vi "Get Standard VI Data.vi"(8 "error in (no error)":errorcluster, 11 "VI Ref":refnum<vi>) -> (0 "error out":errorcluster, 2 "VI Properties":T1, 3 "VI Ref out":refnum<vi>)   [LabVIEW 2020, in "VI Properties Editor.lvlib"]
doc: "Gets all data for a standard VI."
uses:
  VI Properties Editor.lvlib
  <vilib>/picture/picture.llb/imagedata.ctl
  CTLs/VI Properties.ctl
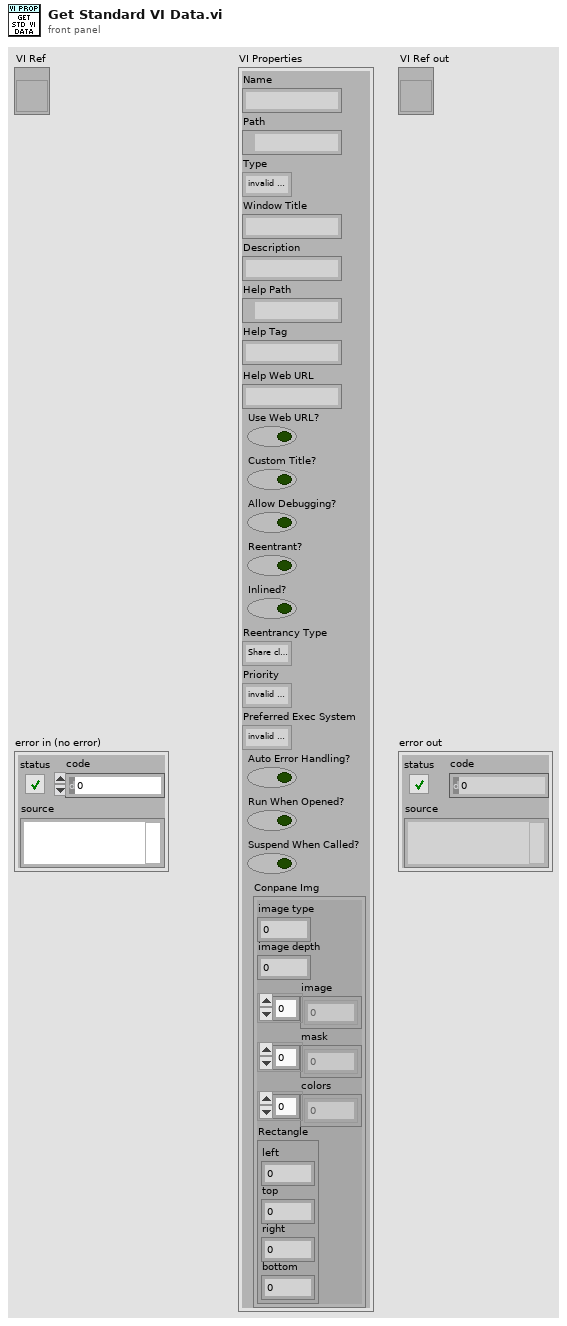
[diagram p1: front panel]
types:
  T1 = typedef "VI Properties Editor.lvlib/VI Properties.ctl" = cluster{"Name":string, "Path":path, "Type":enum32{"invalid VI type", "Standard VI", "Control VI", "Global VI", "Polymorphic VI", "Configuration VI", "SubSystem", "Facade VI", "Method VI", "Statechart Diagram VI"}, "Window Title":string, "Description":string, "Help Path":path, "Help Tag":string, "Help Web URL":string, "Use Web URL?":bool, "Custom Title?":bool, "Allow Debugging?":bool, "Reentrant?":bool, "Inlined?":bool, "Reentrancy Type":enum16{"Share clones between instances", "Preallocate clone for each instance"}, "Priority":enum32{"invalid priority", "background priority", "normal priority", "above normal priority", "high priority", "time critical priority", "subroutine"}, "Preferred Exec System":enum32{"invalid execution system", "user interface", "standard", "instrument i/o", "data acquisition", "other 1", "other 2", "same as caller"}, "Auto Error Handling?":bool, "Run When Opened?":bool, "Suspend When Called?":bool, "Conpane Img":T2}
  T2 = typedef "imagedata.ctl" = cluster{"image type":i32, "image depth":i32, "image":u8[], "mask":u8[], "colors":u32[], "Rectangle":cluster{"left":i16, "top":i16, "right":i16, "bottom":i16}}
  T3 = enum32{"invalid VI type", "Standard VI", "Control VI", "Global VI", "Polymorphic VI", "Configuration VI", "SubSystem", "Facade VI", "Method VI", "Statechart Diagram VI"}
  T4 = enum16{"Share clones between instances", "Preallocate clone for each instance"}
  T5 = enum32{"invalid priority", "background priority", "normal priority", "above normal priority", "high priority", "time critical priority", "subroutine"}
  T6 = enum32{"invalid execution system", "user interface", "standard", "instrument i/o", "data acquisition", "other 1", "other 2", "same as caller"}
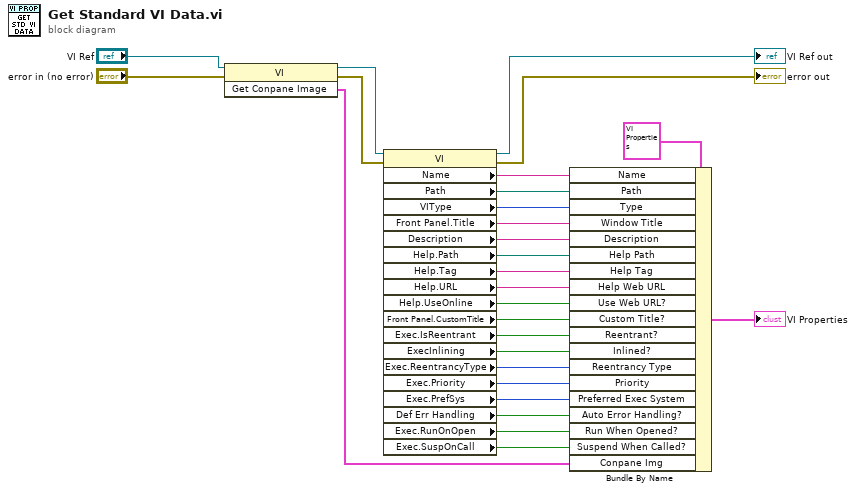
[diagram p0: block diagram]
diagram:
  n1 = invoke class="VI" method="Get Conpane Image"(reference="VI Ref", error in="error in (no error)") -> (reference out=w18:refnum<vi>, error out=w17:errorcluster, "Get Conpane Image"=w1:T2)  [unwired: 1 in]
  n2 = property class="VI"(reference=w18, error in=w17) -> (reference out=→"VI Ref out":refnum<vi>, error out=→"error out":errorcluster, "Name"=w26:string, "Path"=w25:path, "VIType"=w24:T3, "Front Panel.Title"=w13:string, "Description"=w23:string, "Help.Path"=w22:path, "Help.Tag"=w21:string, "Help.URL"=w11:string, "Help.UseOnline"=w10:bool, "Front Panel.CustomTitle"=w12:bool, "Exec.IsReentrant"=w9:bool, "ExecInlining"=w8:bool, "Exec.ReentrancyType"=w7:T4, "Exec.Priority"=w6:T5, "Exec.PrefSys"=w5:T6, "Def Err Handling"=w4:bool, "Exec.RunOnOpen"=w3:bool, "Exec.SuspOnCall"=w2:bool)
  n3 = Bundle By Name(cluster=T1 {"Name"="", "Path"=path "", "Type"=enum."invalid VI type", "Window Title"="", "Description"="", "Help Path"=path "", "Help Tag"="", "Help Web URL"="", "Use Web URL?"=FALSE, "Custom Title?"=FALSE, "Allow Debugging?"=FALSE, "Reentrant?"=FALSE, "Inlined?"=FALSE, "Reentrancy Type"=enum."Share clones between instances", "Priority"=enum."invalid priority", "Preferred Exec System"=enum."invalid execution system", "Auto Error Handling?"=FALSE, "Run When Opened?"=FALSE, "Suspend When Called?"=FALSE, "Conpane Img"={"image type"=0, "image depth"=0, "image"=[], "mask"=[], "colors"=[], "Rectangle"={"left"=0, "top"=0, "right"=0, "bottom"=0}}} ("VI Properties"), "Name"=w26, "Path"=w25, "Type"=w24, "Window Title"=w13, "Description"=w23, "Help Path"=w22, "Help Tag"=w21, "Help Web URL"=w11, "Use Web URL?"=w10, "Custom Title?"=w12, "Reentrant?"=w9, "Inlined?"=w8, "Reentrancy Type"=w7, "Priority"=w6, "Preferred Exec System"=w5, "Auto Error Handling?"=w4, "Run When Opened?"=w3, "Suspend When Called?"=w2, "Conpane Img"=w1) -> (→"VI Properties":T1)
